vi "Teleop.vi"(10 "Match Info":T2={"Autonomous Elapsed Seconds"=0.0, "TeleOp Elapsed Seconds"=138.626, "Disabled Elapsed Seconds"=3.48, "Visited Autonomous"=FALSE, "Visited TeleOp"=TRUE, "Visited Disabled"=TRUE, "Autonomous Settings"={"Autonomous Style"=enum."Independent", "VI Refnum"=refnum}}, 11 "Call Context":T3=enum."Execute") -> ()   [LabVIEW 2017]
doc: "This VI is called for each TeleOp packet received from the DS where the robot is not disabled. It is often used to read from the joysticks and update I/O or to update setpoints for timed control loops. It should complete and return within 20 milliseconds or it may miss DS packets."
uses:
  <vilib>/Rock Robotics/WPI/DriverStation/WPI_DriverStationDerivedRobotMode.ctl
  <vilib>/Rock Robotics/WPI/DriverStation/WPI_DriverStationMatch Info.ctl
  <vilib>/Rock Robotics/WPI/ThirdParty/Phoenix-LabVIEW/Motor Controller/Controls/CTRE_Phoenix_MotorControl_ControlMode.ctl
  <vilib>/Rock Robotics/WPI/Utilities/WPI_GetSetVariantRefNum.vi
  <vilib>/Rock Robotics/Network Tables/NT Write Boolean Array.vi
  <vilib>/Rock Robotics/Network Tables/NT Write Numeric Array.vi
  <vilib>/Rock Robotics/Network Tables/NT Read Boolean.vi
  <vilib>/Rock Robotics/Network Tables/NT Read Number.vi
  <vilib>/Rock Robotics/WPI/ThirdParty/Phoenix-LabVIEW/Motor Controller/Get/CTRE_Phoenix_MotorController_GetSelectedSensorData.vi
  <vilib>/addons/control/pid/NI_PID_pid.lvlib
  <vilib>/addons/control/pid/pid.llb/PID (DBL).vi
  GitHub/FIRST-3958-Controls-Library/NavX/navX Library v2/navX Library v2.lvlib
panel:
  out "Yaw":dbl(graph)
  in  "Angle PID":T1={"proportional gain (Kc)"=1.0, "integral time (Ti, min)"=0.01, "derivative time (Td, min)"=0.0} {"derivative time (Td, min)" format="%.3f"; "integral time (Ti, min)" format="%.3f"; "proportional gain (Kc)" format="%.3f"}
  in  "PID gains 2":T1={"proportional gain (Kc)"=1.0, "integral time (Ti, min)"=0.01, "derivative time (Td, min)"=0.0} {"derivative time (Td, min)" format="%.3f"; "integral time (Ti, min)" format="%.3f"; "proportional gain (Kc)" format="%.3f"}
  in  "y":dbl=1.0
  in  "PID gains":T1={"proportional gain (Kc)"=30.0, "integral time (Ti, min)"=0.01, "derivative time (Td, min)"=0.001} {"derivative time (Td, min)" format="%.3f"; "integral time (Ti, min)" format="%.3f"; "proportional gain (Kc)" format="%.3f"}
  in  "setpoint":dbl format="%.2f"
  out "Position (Raw Sensor Units)":dbl(graph)=-0.000244140625
  out "Sample Slider 0":dbl(slide) scale=0.0..5.0
  out "Sample Boolean 1":bool
  out "Sample Boolean 0":bool
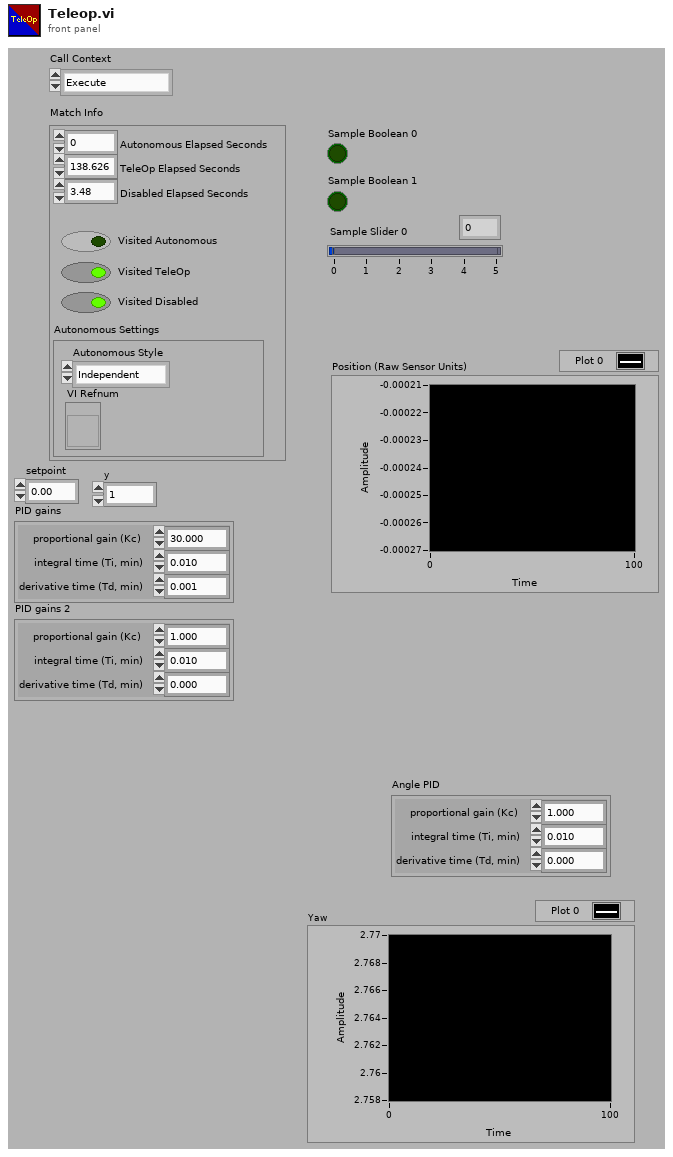
[diagram p1: front panel]
types:
  T1 = cluster{"proportional gain (Kc)":dbl, "integral time (Ti, min)":dbl, "derivative time (Td, min)":dbl}
  T2 = typedef "WPI_DriverStationMatch Info.ctl" = cluster{"Autonomous Elapsed Seconds":dbl, "TeleOp Elapsed Seconds":dbl, "Disabled Elapsed Seconds":dbl, "Visited Autonomous":bool, "Visited TeleOp":bool, "Visited Disabled":bool, "Autonomous Settings":cluster{"Autonomous Style":enum16{"Iterative", "Independent"}, "VI Refnum":refnum<vi>}}
  T3 = typedef "WPI_DriverStationDerivedRobotMode.ctl" = enum16{"Init", "Execute", "Stop"}
  T4 = typedef "CTRE_Phoenix_MotorControl_ControlMode.ctl" = u16
  T5 = typedef "WPI_JoystickDevRef.ctl" = cluster{"Device":T6}
  T6 = typedef "WPI_JoystickDeviceEnum.ctl" = enum16{"USB 0", "USB 1", "USB 2", "USB 3", "USB 4", "USB 5"}
  T7 = typedef "WPI_MotorControlDeviceRef.ctl" = cluster{"DeviceStatus":errorcluster, "Type":T8, "PWM":cluster{"PWM Channel":T9, "DeadBand":T10}, "CAN":cluster{"Device Number":u8, "SetOutput VI Ref":variant, "GetOutput VI Ref":variant, "Enable VI Ref":variant, "Disable VI Ref":variant, "Data":variant}, "Invert":bool, "DIO PWM":cluster{"PWM \"Enable\" Channel":T9, "DIOChannel":T11, "PWM Rate":dbl}}
  T8 = typedef "WPI_MotorControlType.ctl" = enum16{"PWM", "CAN", "DIO PWM"}
  T9 = typedef "FPGA_DIOPWMChannel.ctl" = enum8{"PWM 0", "PWM 1", "PWM 2", "PWM 3", "PWM 4", "PWM 5", "PWM 6", "PWM 7", "PWM 8", "PWM 9", "PWM MXP 0", "PWM MXP 1", "PWM MXP 2", "PWM MXP 3", "PWM MXP 4", "PWM MXP 5", "PWM MXP 6", "PWM MXP 7", "PWM MXP 8", "PWM MXP 9", "Invalid"}
  T10 = typedef "WPI_PWMDeadband.ctl" = cluster{"Name":string, "maxPositivePwm":i32, "minPositivePwm":i32, "centerPwm":i32, "maxNegativePwm":i32, "minNegativePwm":i32, "angularRange":u16}
  T11 = typedef "FPGA_DIOChannel.ctl" = enum8{"DIO 0", "DIO 1", "DIO 2", "DIO 3", "DIO 4", "DIO 5", "DIO 6", "DIO 7", "DIO 8", "DIO 9", "DIO MXP 0", "DIO MXP 1", "DIO MXP 2", "DIO MXP 3", "DIO MXP 4", "DIO MXP 5", "DIO MXP 6", "DIO MXP 7", "DIO MXP 8", "DIO MXP 9", "DIO MXP 10", "DIO MXP 11", "DIO MXP 12", "DIO MXP 13", "DIO MXP 14", "DIO MXP 15", "SPI Port CS1", "SPI Port CS2", "SPI Port CS3", "SPI Port MISO", "SPI Port MOSI", "Invalid"}
  T12 = typedef "navX Library v2.lvlib/Z900_navX_DeviceTypeDef.ctl" = cluster{"Interface":cluster{"Protocol":T13, "Update Rate (4Hz-100Hz)":u8, "navX Open TypeDef":variant}, "Notify Packet":refnum<notifier>, "Loop VI Refnum":refnum<vi>, "Ready to Close Occurrence Refnum":refnum<k4>}
  T13 = typedef "navX Library v2.lvlib/Z900_navX_ProtocolTypeDef.ctl" = enum16{"SERIAL", "I2C", "SPI"}
  T14 = cluster{"Yaw":dbl, "Roll":dbl, "Pitch":dbl, "Heading":dbl, "Fused Heading":dbl}
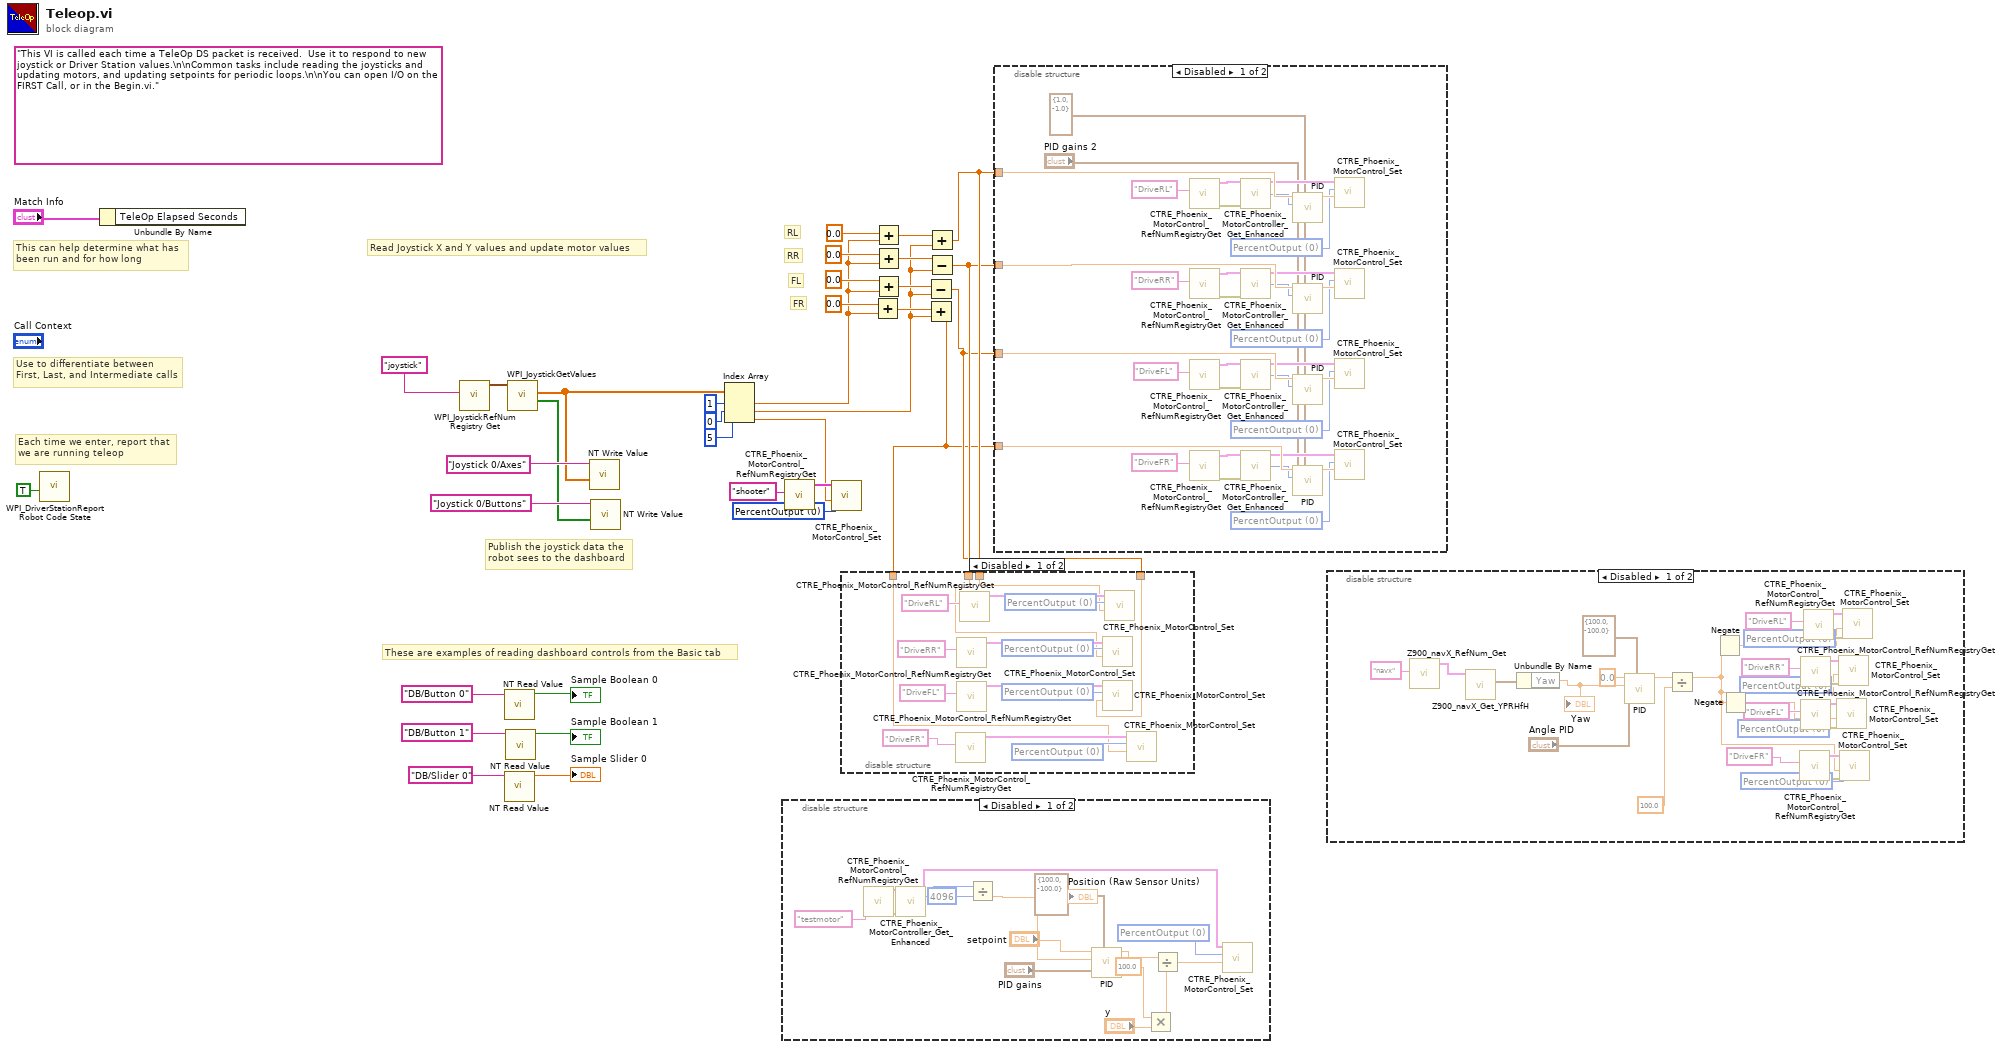
[diagram p0: block diagram]
diagram:
  w2 = T4 0 items=["PercentOutput"=0, "Position"=1, "Velocity"=2, "Current"=3, "Follower"=5, "MotionProfile"=6, "MotionMagic"=7, "MotionMagicArc"=8, "MotionProfileArc"=10, "Disabled"=15] ("Control Mode")
  (unwired) "This VI is called each time a TeleOp DS packet is received.  Use it to respond to new joystick or Driver Station values.\n\nCommon tasks include reading the joysticks and updating motors, and updating setpoints for periodic loops.\n\nYou can open I/O on the FIRST Call, or in the Begin.vi."
  # "FR"
  # "FL"
  # "RR"
  # "RL"
  # "These are examples of reading dashboard controls from the Basic tab"
  # "Publish the joystick data the\nrobot sees to the dashboard"
  # "Each time we enter, report that\nwe are running teleop"
  # "Use to differentiate between\nFirst, Last, and Intermediate calls"
  # "This can help determine what has\nbeen run and for how long"
  # "Read Joystick X and Y values and update motor values"
  n1 = call <vilib>:"WPI_DriverStationReport Robot Code State.vi"("TeleOp"=TRUE ("Autonomous")) -> ()  [unwired: 10 in, 1 out]
  n2 = Unbundle By Name("Match Info") -> ()  [unwired: 1 out]
  n3 = call <vilib>:"WPI_JoystickRefNum Registry Get.vi"("refnum name"="joystick") -> ("JoystickDevRef"=w33:T5)  [unwired: 1 in, 9 out]
  n4 = call-poly <vilib>:"NT Read Value.vi"("Name"="DB/Button 0" ("refnum name")) -> ("Boolean"=→"Sample Boolean 0":bool)  [unwired: 9 in, 1 out]
  n5 = call-poly <vilib>:"NT Read Value.vi"("Name"="DB/Slider 0" ("refnum name")) -> ("Numeric"=→"Sample Slider 0":dbl)  [unwired: 9 in, 1 out]
  n6 = call-poly <vilib>:"NT Read Value.vi"("Name"="DB/Button 1" ("refnum name")) -> ("Boolean"=→"Sample Boolean 1":bool)  [unwired: 9 in, 1 out]
  n7 = call <vilib>:"WPI_JoystickGetValues.vi"("JoystickDevRef"=w33) -> ("Buttons"=w29:bool[], "Axes"=w22:dbl[])  [unwired: 6 in, 3 out]
  n8 = call-poly <vilib>:"NT Write Value.vi"("Numeric Array"=w22, "Name"="Joystick 0/Axes") -> ()  [unwired: 9 in, 1 out]
  n9 = call-poly <vilib>:"NT Write Value.vi"("Boolean Array"=w29, "Name"="Joystick 0/Buttons") -> ()  [unwired: 9 in, 1 out]
  n10 = Index Array(array=w22, index #1=1 ("index"), index #2=0 ("index"), index #3=5 ("index")) -> (element #1=w17:dbl, element #2=w12:dbl, element #3=w1:dbl)
  n11 = disable-structure shown="Disabled" {
    frame Disabled {
      w39 = T4 0 items=["PercentOutput"=0, "Position"=1, "Velocity"=2, "Current"=3, "Follower"=5, "MotionProfile"=6, "MotionMagic"=7, "MotionMagicArc"=8, "MotionProfileArc"=10, "Disabled"=15] ("Control Mode")
      n12 = call <vilib>:"CTRE_Phoenix_MotorControl_RefNumRegistryGet.vi"("refnum name"="testmotor") -> ("error out"=w50:errorcluster, "PhoenixMotorControlDevRef"=w51:T7)  [unwired: 9 in]
      n13 = call-poly <vilib>:"CTRE_Phoenix_MotorController_Get_Enhanced.vi"("PhoenixMotorControlDevRef"=w51, "error in"=w50) -> ("PhoenixMotorControlDevRef"=w38:T7, "Position (Raw Sensor Units)"=w48:i32)  [unwired: 10 in, 2 out]
      n14 = Divide(x=w48, y=4096) -> (x/y=w46:dbl)
      "Position (Raw Sensor Units)" <- w46
      n15 = call-poly <vilib>:"PID.vi"("output range"=cluster{"output high":dbl, "output low":dbl} {"output high"=100.0, "output low"=-100.0}, "PID gains"="PID gains", "process variable"=w46, "setpoint"="setpoint") -> ("output"=w42:dbl)  [unwired: 6 in, 1 out]
      n16 = Multiply(x=100.0 ("y"), y="y") -> (x*y=w37:dbl)
      n17 = Divide(x=w42, y=w37) -> (x/y=w40:dbl)
      n18 = call <vilib>:"CTRE_Phoenix_MotorControl_Set.vi"("Output"=w40, "Control Mode"=w39, "PhoenixMotorControlDevRef"=w38) -> ()  [unwired: 7 in, 2 out]
    }
    frame Enabled {
    }
  }
  n19 = call <vilib>:"CTRE_Phoenix_MotorControl_RefNumRegistryGet.vi"("refnum name"="shooter") -> ("PhoenixMotorControlDevRef"=w3:T7)  [unwired: 9 in, 1 out]
  n20 = call <vilib>:"CTRE_Phoenix_MotorControl_Set.vi"("Output"=w1, "Control Mode"=w2, "PhoenixMotorControlDevRef"=w3) -> ()  [unwired: 7 in, 2 out]
  n21 = Add(x=0.0, y=w17) -> (x+y=w15:dbl)
  n22 = Add(x=0.0, y=w17) -> (x+y=w16:dbl)
  n23 = Add(x=0.0, y=w17) -> (x+y=w14:dbl)
  n24 = Add(x=0.0, y=w17) -> (x+y=w13:dbl)
  n25 = Subtract(x=w13, y=w12) -> (x-y=w7:dbl)
  n26 = Add(x=w15, y=w12) -> (x+y=w6:dbl)
  n27 = Add(x=w16, y=w12) -> (x+y=w9:dbl)
  n28 = Subtract(x=w14, y=w12) -> (x-y=w8:dbl)
  n29 = disable-structure shown="Disabled" {
    disable-tunnel: w9 -> [w55 _]
    disable-tunnel: w8 -> [w54 _]
    disable-tunnel: w7 -> [w53 _]
    disable-tunnel: w6 -> [w52 _]
    frame Disabled {
      w56 = T4 0 items=["PercentOutput"=0, "Position"=1, "Velocity"=2, "Current"=3, "Follower"=5, "MotionProfile"=6, "MotionMagic"=7, "MotionMagicArc"=8, "MotionProfileArc"=10, "Disabled"=15] ("Control Mode")
      w59 = T4 0 items=["PercentOutput"=0, "Position"=1, "Velocity"=2, "Current"=3, "Follower"=5, "MotionProfile"=6, "MotionMagic"=7, "MotionMagicArc"=8, "MotionProfileArc"=10, "Disabled"=15] ("Control Mode")
      w62 = T4 0 items=["PercentOutput"=0, "Position"=1, "Velocity"=2, "Current"=3, "Follower"=5, "MotionProfile"=6, "MotionMagic"=7, "MotionMagicArc"=8, "MotionProfileArc"=10, "Disabled"=15] ("Control Mode")
      w65 = T4 0 items=["PercentOutput"=0, "Position"=1, "Velocity"=2, "Current"=3, "Follower"=5, "MotionProfile"=6, "MotionMagic"=7, "MotionMagicArc"=8, "MotionProfileArc"=10, "Disabled"=15] ("Control Mode")
      n30 = call <vilib>:"CTRE_Phoenix_MotorControl_RefNumRegistryGet.vi"("refnum name"="DriveFR") -> ("PhoenixMotorControlDevRef"=w60:T7)  [unwired: 9 in, 1 out]
      n31 = call <vilib>:"CTRE_Phoenix_MotorControl_RefNumRegistryGet.vi"("refnum name"="DriveRR") -> ("PhoenixMotorControlDevRef"=w57:T7)  [unwired: 9 in, 1 out]
      n32 = call <vilib>:"CTRE_Phoenix_MotorControl_RefNumRegistryGet.vi"("refnum name"="DriveFL") -> ("PhoenixMotorControlDevRef"=w63:T7)  [unwired: 9 in, 1 out]
      n33 = call <vilib>:"CTRE_Phoenix_MotorControl_RefNumRegistryGet.vi"("refnum name"="DriveRL") -> ("PhoenixMotorControlDevRef"=w66:T7)  [unwired: 9 in, 1 out]
      n34 = call <vilib>:"CTRE_Phoenix_MotorControl_Set.vi"("Output"=w54, "Control Mode"=w56, "PhoenixMotorControlDevRef"=w57) -> ()  [unwired: 7 in, 2 out]
      n35 = call <vilib>:"CTRE_Phoenix_MotorControl_Set.vi"("Output"=w53, "Control Mode"=w62, "PhoenixMotorControlDevRef"=w63) -> ()  [unwired: 7 in, 2 out]
      n36 = call <vilib>:"CTRE_Phoenix_MotorControl_Set.vi"("Output"=w55, "Control Mode"=w65, "PhoenixMotorControlDevRef"=w66) -> ()  [unwired: 7 in, 2 out]
      n37 = call <vilib>:"CTRE_Phoenix_MotorControl_Set.vi"("Output"=w52, "Control Mode"=w59, "PhoenixMotorControlDevRef"=w60) -> ()  [unwired: 7 in, 2 out]
    }
    frame Enabled {
    }
  }
  n38 = disable-structure shown="Disabled" {
    disable-tunnel: w6 -> [w101 _]
    disable-tunnel: w7 -> [w100 _]
    disable-tunnel: w8 -> [w99 _]
    disable-tunnel: w9 -> [w98 _]
    frame Disabled {
      w69 = cluster{"output high":dbl, "output low":dbl} {"output high"=1.0, "output low"=-1.0} ("output range")
      w70 = T4 0 items=["PercentOutput"=0, "Position"=1, "Velocity"=2, "Current"=3, "Follower"=5, "MotionProfile"=6, "MotionMagic"=7, "MotionMagicArc"=8, "MotionProfileArc"=10, "Disabled"=15] ("Control Mode")
      w71 = T4 0 items=["PercentOutput"=0, "Position"=1, "Velocity"=2, "Current"=3, "Follower"=5, "MotionProfile"=6, "MotionMagic"=7, "MotionMagicArc"=8, "MotionProfileArc"=10, "Disabled"=15] ("Control Mode")
      w72 = T4 0 items=["PercentOutput"=0, "Position"=1, "Velocity"=2, "Current"=3, "Follower"=5, "MotionProfile"=6, "MotionMagic"=7, "MotionMagicArc"=8, "MotionProfileArc"=10, "Disabled"=15] ("Control Mode")
      w73 = T4 0 items=["PercentOutput"=0, "Position"=1, "Velocity"=2, "Current"=3, "Follower"=5, "MotionProfile"=6, "MotionMagic"=7, "MotionMagicArc"=8, "MotionProfileArc"=10, "Disabled"=15] ("Control Mode")
      n39 = call <vilib>:"CTRE_Phoenix_MotorControl_RefNumRegistryGet.vi"("refnum name"="DriveRL") -> ("error out"=w94:errorcluster, "PhoenixMotorControlDevRef"=w95:T7)  [unwired: 9 in]
      n40 = call <vilib>:"CTRE_Phoenix_MotorControl_RefNumRegistryGet.vi"("refnum name"="DriveRR") -> ("error out"=w92:errorcluster, "PhoenixMotorControlDevRef"=w93:T7)  [unwired: 9 in]
      n41 = call <vilib>:"CTRE_Phoenix_MotorControl_RefNumRegistryGet.vi"("refnum name"="DriveFL") -> ("error out"=w91:errorcluster, "PhoenixMotorControlDevRef"=w90:T7)  [unwired: 9 in]
      n42 = call <vilib>:"CTRE_Phoenix_MotorControl_RefNumRegistryGet.vi"("refnum name"="DriveFR") -> ("error out"=w88:errorcluster, "PhoenixMotorControlDevRef"=w89:T7)  [unwired: 9 in]
      n43 = call-poly <vilib>:"CTRE_Phoenix_MotorController_Get_Enhanced.vi"("PhoenixMotorControlDevRef"=w95, "error in"=w94) -> ("PhoenixMotorControlDevRef"=w77:T7, "Velocity (Raw Sensor Units per 100 ms)"=w85:i32)  [unwired: 10 in, 2 out]
      n44 = call-poly <vilib>:"CTRE_Phoenix_MotorController_Get_Enhanced.vi"("PhoenixMotorControlDevRef"=w93, "error in"=w92) -> ("PhoenixMotorControlDevRef"=w76:T7, "Velocity (Raw Sensor Units per 100 ms)"=w84:i32)  [unwired: 10 in, 2 out]
      n45 = call-poly <vilib>:"CTRE_Phoenix_MotorController_Get_Enhanced.vi"("PhoenixMotorControlDevRef"=w90, "error in"=w91) -> ("PhoenixMotorControlDevRef"=w75:T7, "Velocity (Raw Sensor Units per 100 ms)"=w83:i32)  [unwired: 10 in, 2 out]
      n46 = call-poly <vilib>:"CTRE_Phoenix_MotorController_Get_Enhanced.vi"("PhoenixMotorControlDevRef"=w89, "error in"=w88) -> ("PhoenixMotorControlDevRef"=w74:T7, "Velocity (Raw Sensor Units per 100 ms)"=w82:i32)  [unwired: 10 in, 2 out]
      n47 = call-poly <vilib>:"PID.vi"("output range"=w69, "PID gains"="PID gains 2", "process variable"=w85, "setpoint"=w98) -> ("output"=w81:dbl)  [unwired: 6 in, 1 out]
      n48 = call-poly <vilib>:"PID.vi"("output range"=w69, "PID gains"="PID gains 2", "process variable"=w84, "setpoint"=w99) -> ("output"=w80:dbl)  [unwired: 6 in, 1 out]
      n49 = call-poly <vilib>:"PID.vi"("output range"=w69, "PID gains"="PID gains 2", "process variable"=w83, "setpoint"=w100) -> ("output"=w79:dbl)  [unwired: 6 in, 1 out]
      n50 = call-poly <vilib>:"PID.vi"("output range"=w69, "PID gains"="PID gains 2", "process variable"=w82, "setpoint"=w101) -> ("output"=w78:dbl)  [unwired: 6 in, 1 out]
      n51 = call <vilib>:"CTRE_Phoenix_MotorControl_Set.vi"("Output"=w81, "Control Mode"=w73, "PhoenixMotorControlDevRef"=w77) -> ()  [unwired: 7 in, 2 out]
      n52 = call <vilib>:"CTRE_Phoenix_MotorControl_Set.vi"("Output"=w80, "Control Mode"=w72, "PhoenixMotorControlDevRef"=w76) -> ()  [unwired: 7 in, 2 out]
      n53 = call <vilib>:"CTRE_Phoenix_MotorControl_Set.vi"("Output"=w79, "Control Mode"=w71, "PhoenixMotorControlDevRef"=w75) -> ()  [unwired: 7 in, 2 out]
      n54 = call <vilib>:"CTRE_Phoenix_MotorControl_Set.vi"("Output"=w78, "Control Mode"=w70, "PhoenixMotorControlDevRef"=w74) -> ()  [unwired: 7 in, 2 out]
    }
    frame Enabled {
    }
  }
  n55 = disable-structure shown="Disabled" {
    frame Disabled {
      w110 = T4 0 items=["PercentOutput"=0, "Position"=1, "Velocity"=2, "Current"=3, "Follower"=5, "MotionProfile"=6, "MotionMagic"=7, "MotionMagicArc"=8, "MotionProfileArc"=10, "Disabled"=15] ("Control Mode")
      w111 = T4 0 items=["PercentOutput"=0, "Position"=1, "Velocity"=2, "Current"=3, "Follower"=5, "MotionProfile"=6, "MotionMagic"=7, "MotionMagicArc"=8, "MotionProfileArc"=10, "Disabled"=15] ("Control Mode")
      w112 = T4 0 items=["PercentOutput"=0, "Position"=1, "Velocity"=2, "Current"=3, "Follower"=5, "MotionProfile"=6, "MotionMagic"=7, "MotionMagicArc"=8, "MotionProfileArc"=10, "Disabled"=15] ("Control Mode")
      w113 = T4 0 items=["PercentOutput"=0, "Position"=1, "Velocity"=2, "Current"=3, "Follower"=5, "MotionProfile"=6, "MotionMagic"=7, "MotionMagicArc"=8, "MotionProfileArc"=10, "Disabled"=15] ("Control Mode")
      n56 = call "Z900_navX_RefNum_Get.vi"("refnum name"="navx") -> ("navX Device"=w103:T12)  [unwired: 9 in, 1 out]
      n57 = call "Z900_navX_Get_YPRHfH.vi"("navX Device"=w103) -> ("YRPHfH"=w102:T14)  [unwired: 7 in, 3 out]
      n58 = Unbundle By Name(w102) -> ("Yaw"=w129:dbl)
      "Yaw" <- w129
      n59 = call-poly <vilib>:"PID.vi"("output range"=cluster{"output high":dbl, "output low":dbl} {"output high"=100.0, "output low"=-100.0}, "PID gains"="Angle PID", "process variable"=w129, "setpoint"=0.0) -> ("output"=w107:dbl)  [unwired: 6 in, 1 out]
      n60 = Divide(x=w107, y=100.0) -> (x/y=w106:dbl)
      n61 = Negate(x=w106) -> (-x=w109:dbl)
      n62 = Negate(x=w106) -> (-x=w108:dbl)
      n63 = call <vilib>:"CTRE_Phoenix_MotorControl_RefNumRegistryGet.vi"("refnum name"="DriveFR") -> ("error out"=w115:errorcluster, "PhoenixMotorControlDevRef"=w114:T7)  [unwired: 9 in]
      n64 = call <vilib>:"CTRE_Phoenix_MotorControl_RefNumRegistryGet.vi"("refnum name"="DriveRR") -> ("error out"=w119:errorcluster, "PhoenixMotorControlDevRef"=w118:T7)  [unwired: 9 in]
      n65 = call <vilib>:"CTRE_Phoenix_MotorControl_RefNumRegistryGet.vi"("refnum name"="DriveFL") -> ("error out"=w117:errorcluster, "PhoenixMotorControlDevRef"=w116:T7)  [unwired: 9 in]
      n66 = call <vilib>:"CTRE_Phoenix_MotorControl_RefNumRegistryGet.vi"("refnum name"="DriveRL") -> ("error out"=w121:errorcluster, "PhoenixMotorControlDevRef"=w120:T7)  [unwired: 9 in]
      n67 = call <vilib>:"CTRE_Phoenix_MotorControl_Set.vi"("error in (no error)"=w117, "Output"=w108, "Control Mode"=w112, "PhoenixMotorControlDevRef"=w116) -> ()  [unwired: 6 in, 2 out]
      n68 = call <vilib>:"CTRE_Phoenix_MotorControl_Set.vi"("error in (no error)"=w119, "Output"=w106, "Control Mode"=w111, "PhoenixMotorControlDevRef"=w118) -> ()  [unwired: 6 in, 2 out]
      n69 = call <vilib>:"CTRE_Phoenix_MotorControl_Set.vi"("error in (no error)"=w115, "Output"=w106, "Control Mode"=w113, "PhoenixMotorControlDevRef"=w114) -> ()  [unwired: 6 in, 2 out]
      n70 = call <vilib>:"CTRE_Phoenix_MotorControl_Set.vi"("error in (no error)"=w121, "Output"=w109, "Control Mode"=w110, "PhoenixMotorControlDevRef"=w120) -> ()  [unwired: 6 in, 2 out]
    }
    frame Enabled {
    }
  }
